vi "Get Node Incoming Edges.vi"(10 "Node":variant, 11 "Abstract Graph in":refnum<class "Abstract Graph.lvclass">) -> (1 "Node Exist":bool, 2 "Incoming Edges":T1[](array[typedef]), 3 "Abstract Graph out":refnum<class "Abstract Graph.lvclass">)   [LabVIEW 2021, in "GraphLib.lvlib" / "Directed Graph.lvclass"]
uses:
  Directed Graph/Directed Graph.lvclass
  Directed Graph/Directed Graph.lvclass/Directed Graph.ctl
  Abstract Graph.lvclass
  Edge.ctl
  GraphLib.lvlib
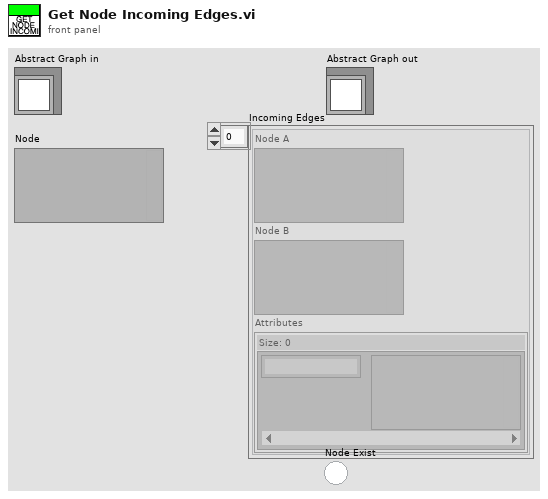
[diagram p1: front panel]
types:
  T1 = typedef "GraphLib.lvlib/Edge.ctl" = cluster{"Node A":variant, "Node B":variant, "Attributes":map{string, variant}}
  T2 = typedef "GraphLib.lvlib/Cluster - Graph Node.ctl" = cluster{"Value":variant, "Child Node IDs":set{string}, "Attributes":map{string, string}}
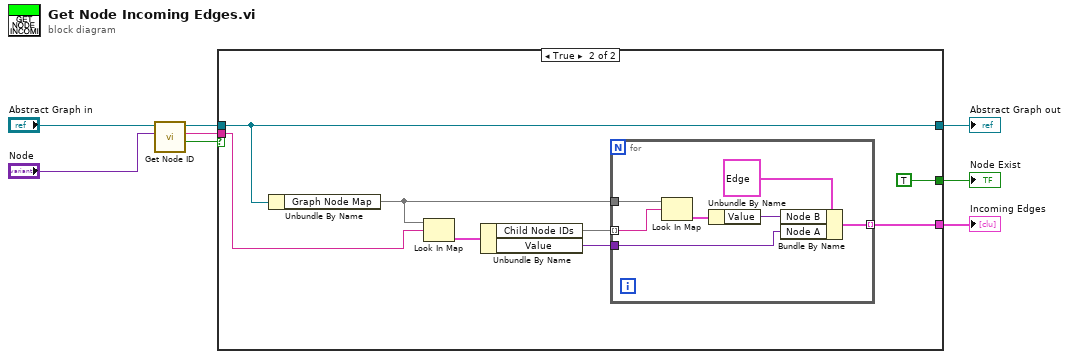
[diagram p0: block diagram]
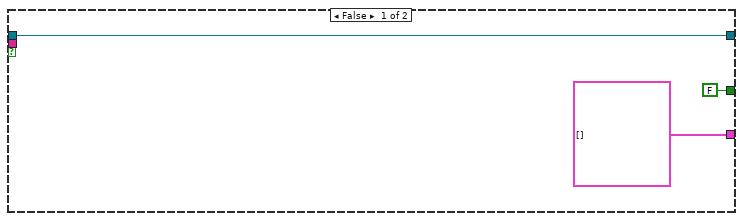
[diagram p2: hidden frame]
diagram:
  n1 = call "Get Node ID.vi"("Node"="Node", "Abstract Graph in"="Abstract Graph in") -> ("Node Exist"=w6:bool, "Node ID"=w4:string, "Abstract Graph out"=w5:refnum<class "Abstract Graph.lvclass">)  [unwired: 7 in]
  n2 = case shown="True" w6 {
    tunnel: w5 -> [w9 w13]
    tunnel: w4 -> [_ w19]
    tunnel: [T1[] [] w14] -> w3
    tunnel: [w9 w13] -> w2
    tunnel: [FALSE TRUE] -> w1
    frame False {
    }
    frame True {
      n3 = Unbundle By Name(w13) -> ("Graph Node Map"=w17)
      n4 = Look In Map(map=w17, key=w19) -> (value=w18:T2)  [unwired: 1 in, 1 out]
      n5 = Unbundle By Name(w18) -> ("Child Node IDs"=w16:set{string}, "Value"=w15:variant)
      n6 = for {
        tunnel: w17 -> [w26]
        tunnel: w16 -> [w25] mode=indexing
        tunnel: w15 -> [w21]
        tunnel: [w20] -> w14 mode=indexing
        n7 = Look In Map(map=w26, key=w25) -> (value=w24:T2)  [unwired: 1 in, 1 out]
        n8 = Unbundle By Name(w24) -> ("Value"=w22:variant)
        n9 = Bundle By Name(cluster=T1 {"Node A"=variant, "Node B"=variant, "Attributes"={}} ("Cluster - Edge"), "Node B"=w22, "Node A"=w21) -> (w20:T1)
      }
    }
  }
  "Abstract Graph out" <- w2
  "Incoming Edges" <- w3
  "Node Exist" <- w1
